vi "Write Number of Tatics.vi"(8 "error in (no error)":errorcluster, 10 "Number of Tatics":dbl=1.0, 11 "5RobotsRole in":refnum<class "5RobotsRole.lvclass">) -> (0 "error out":errorcluster, 3 "5RobotsRole out":refnum<class "5RobotsRole.lvclass">)   [LabVIEW 2020, in "5RobotsRole.lvclass"]
uses:
  5RobotsRole.lvclass
  5RobotsRole.lvclass/5RobotsRole.ctl
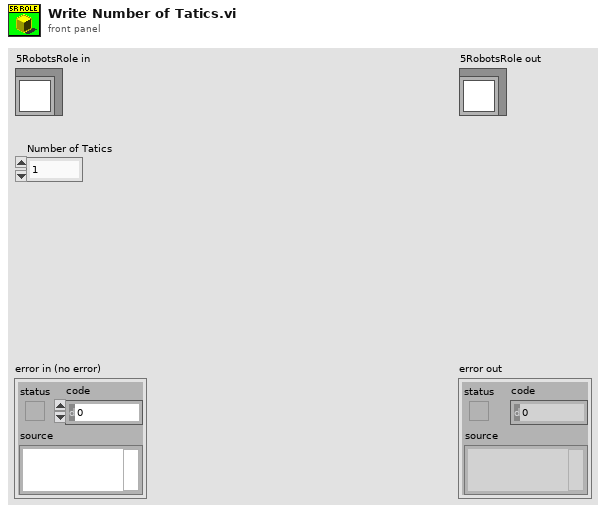
[diagram p1: front panel]
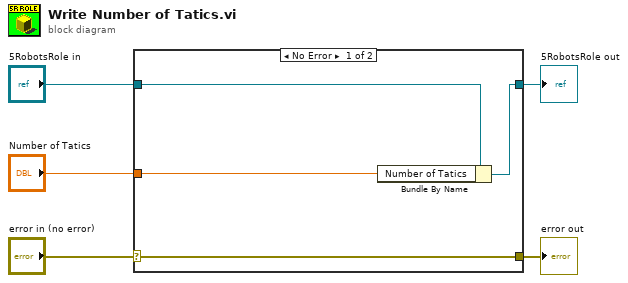
[diagram p0: block diagram]
diagram:
  n1 = case shown="No Error" "error in (no error)" {
    selector: "error in (no error)" -> [w9 w10]
    tunnel: [w9 w10] -> w4
    tunnel: [w7 w11] -> w2
    tunnel: "5RobotsRole in" -> [w8 w11]
    tunnel: "Number of Tatics" -> [w6 _]
    frame No Error {
      n2 = Bundle By Name(cluster=w8, "Number of Tatics"=w6) -> (w7:refnum<class "5RobotsRole.lvclass">)
    }
    frame Error {
    }
  }
  "error out" <- w4
  "5RobotsRole out" <- w2
